vi "Ramsete Command.vi"(7 "Trackwidth":dbl, 8 "Reset? (F)":bool, 9 "timestamp (s)":dbl, 10 "Trajectory":T4[](array[typedef]), 11 "Pose2d":T1) -> (1 "Finished?":bool, 2 "Right Velocity Ref":dbl, 3 "Left Velocity Ref":dbl)   [LabVIEW 2019]
uses:
  <vilib>/Rock Robotics/WPI/ThirdParty/WPILib Extensions/Trajectory/Typedef/Trajectory State.ctl
  <vilib>/Rock Robotics/WPI/ThirdParty/WPILib Extensions/Geometry/Typedef/Pose2d.ctl
  <vilib>/Rock Robotics/WPI/ThirdParty/WPILib Extensions/Geometry/Typedef/Translation2d.ctl
  <vilib>/Rock Robotics/WPI/ThirdParty/WPILib Extensions/Geometry/Typedef/Rotation2d.ctl
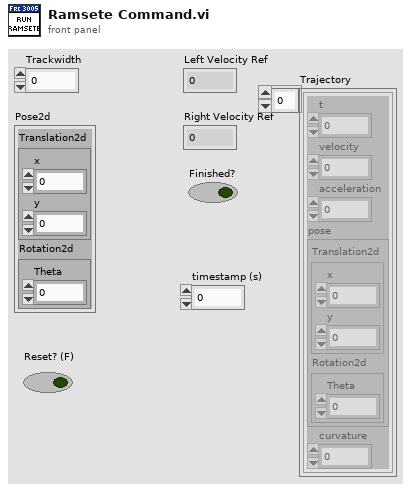
[diagram p1: front panel]
types:
  T1 = typedef "Pose2d.ctl" = cluster{"Translation2d":T2, "Rotation2d":T3}
  T2 = typedef "Translation2d.ctl" = cluster{"x":dbl, "y":dbl}
  T3 = typedef "Rotation2d.ctl" = cluster{"Theta":dbl}
  T4 = typedef "Trajectory State.ctl" = cluster{"t":dbl, "velocity":dbl, "acceleration":dbl, "pose":T1, "curvature":dbl}
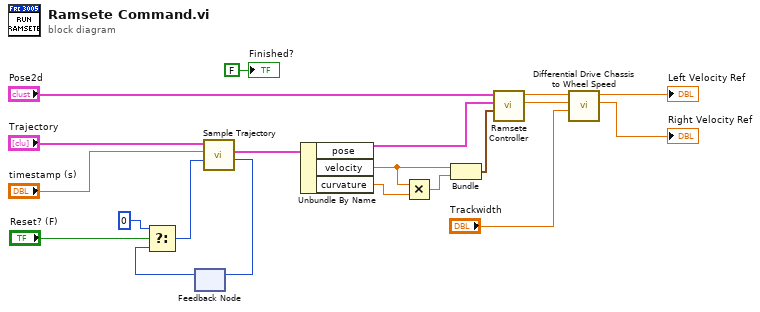
[diagram p0: block diagram]
diagram:
  n1 = feedback #1() -> (w7:i32)  [unwired: 1 in]
  n2 = Select(t=0, s="Reset? (F)", f=w7) -> (s? t:f=w5:i32)
  n3 = call <vilib>:"Sample Trajectory.vi"("start index (0)"=w5, "timestamp (s)"="timestamp (s)", "Trajectory States"="Trajectory") -> ("index"=w8:i32, "State"=w15:T4)  [unwired: 6 in, 1 out]
  n4 = feedback-in #1(w8) -> ()
  n5 = Unbundle By Name(w15) -> ("pose"=w16:T1, "velocity"=w18:dbl, "curvature"=w19:dbl)
  n6 = Multiply(x=w18, y=w19) -> (x*y=w17:dbl)
  n7 = Bundle("velocity"=w18, w17) -> (w20:cluster{"velocity":dbl, dbl})  [unwired: 1 in]
  n8 = call <vilib>:"Ramsete Controller.vi"("Velocity Ref"=w20, "Pose Ref"=w16, "Current Pose"="Pose2d") -> ("Angular Velocity"=w12:dbl, "Linear Velocity"=w11:dbl)  [unwired: 7 in]
  n9 = call <vilib>:"Differential Drive Chassis to Wheel Speed.vi"("Trackwidth"="Trackwidth", "Angular Velocity"=w12, "Linear Velocity"=w11) -> ("right"=→"Right Velocity Ref":dbl, "left"=→"Left Velocity Ref":dbl)  [unwired: 7 in]
  "Finished?" <- FALSE ("Finished?")
